vi "Write Meta Value.vi"(8 "error in (no error)":errorcluster, 9 "Meta Value":string, 10 "Meta Name":string, 11 "Config Element in":refnum<class "Config Element.lvclass">) -> (0 "error out":errorcluster, 3 "Config Element out":refnum<class "Config Element.lvclass">)   [LabVIEW 2023, in "CDM-Config.lvlib" / "Config Element.lvclass"]
doc: "Writes a single meta value to the element. If the meta field already exists with the specified name, the value will be updated to the new value."
uses:
  Config Element.lvclass
  Config Element.lvclass/Config Element.ctl
  Meta Data.ctl
  CDM-Config.lvlib
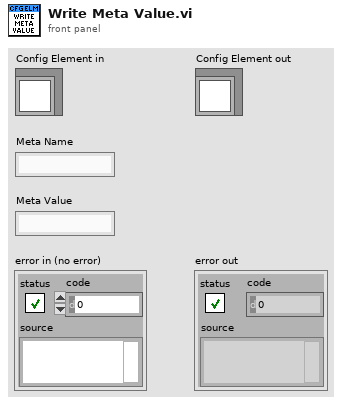
[diagram p1: front panel]
types:
  T1 = typedef "CDM-Config.lvlib/Meta Data.ctl" = cluster{"Name":string, "Value":string}
  T2 = typedef "CDM-Config.lvlib/Config Element.lvclass/Element Data.ctl" = cluster{"Node Info":T3, "Owner":refnum<class>, "Changed":bool, "Name":string, "Meta Data":T1[], "Value Type":T4, "Value":variant}
  T3 = typedef "CDM-Config.lvlib/Node Info.ctl" = cluster{"Index":i32, "Parent":i32, "Children":i32[]}
  T4 = typedef "CDM-Config.lvlib/Value Type.ctl" = enum16{"String", "Number", "Bool", "Object", "Array"}
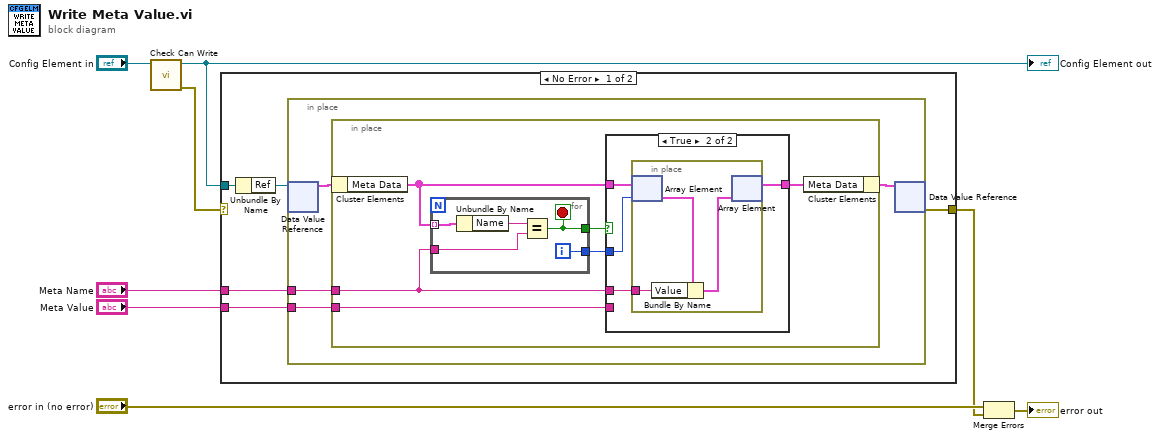
[diagram p0: block diagram]
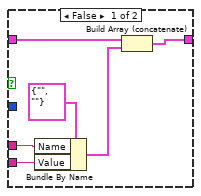
[diagram p2: hidden frame]
diagram:
  n1 = call "Check Can Write.vi"("Config Element in"="Config Element in") -> ("error out"=w1:errorcluster, "Config Element out"=w2:refnum<class "Config Element.lvclass">)  [unwired: 9 in]
  "Config Element out" <- w2
  n2 = case shown="No Error" w1 {
    selector: w1 -> [_ w42]
    tunnel: "Meta Name" -> [w12 _]
    tunnel: "Meta Value" -> [w11 _]
    tunnel: [w10 w42] -> w3
    tunnel: w2 -> [w9 _]
    frame No Error {
      n3 = Unbundle By Name(w9) -> ("Ref"=w13:refnum<data-value>)
      n4 = in-place {
        in-place-border: w12 -> [w15]
        in-place-border: w11 -> [w14]
        n5 = in-place-dvr #1(w13) -> (w17:T2)  [unwired: 1 out]
        n6 = in-place {
          in-place-border: w15 -> [w21]
          in-place-border: w14 -> [w18]
          n7 = in-place-cluster #2(w17) -> ("Meta Data"=w23:T1[])
          n8 = for {
            tunnel: w23 -> [w41] mode=indexing
            tunnel: w21 -> [w39]
            tunnel: [w38] -> w20
            tunnel: [w37] -> w19
            i -> [w37]
            stop <- w38 stop-if-true
            n9 = Unbundle By Name(w41) -> ("Name"=w40:string)
            n10 = Equal?(x=w40, y=w39) -> (x = y?=w38:bool)
          }
          n11 = case shown="True" w20 {
            tunnel: w19 -> [_ w31]
            tunnel: w23 -> [w29 w32]
            tunnel: w21 -> [w26 w33]
            tunnel: [w28 w30] -> w22
            tunnel: w18 -> [w25 _]
            frame False {
              n12 = Bundle By Name(cluster=T1 {"Name"="", "Value"=""} ("Meta Data"), "Name"=w26, "Value"=w25) -> (w24:T1)
              n13 = Build Array (concatenate)(w29, w24) -> (w28:T1[])
            }
            frame True {
              n14 = in-place {
                in-place-border: w33 -> [w35]
                n15 = in-place-array #3(w32, w31) -> (w36:T1)
                n16 = Bundle By Name(cluster=w36, "Value"=w35) -> (w34:T1)
                n17 = in-place-array #3(w34) -> (w30:T1[])  [unwired: 1 out]
              }
            }
          }
          n18 = in-place-cluster #2("Meta Data"=w22) -> (w16:T2)
        }
        n19 = in-place-dvr #1(w16) -> (w10:errorcluster)  [unwired: 1 out]
      }
    }
    frame Error {
    }
  }
  n20 = Merge Errors("error in (no error)", w3) -> (→"error out":errorcluster)
